vi "scanToString.vi"(0 "instrument handle":refnum<k15>, 1 "wfm info":T3(array[cluster]), 2 "Immediate Trigger Received":bool, 4 "Channels and coupling":T1, 5 "wfm":i8[][](array[numeric]), 9 "Triger Source":i32, 11 "error in":errorcluster {"code" format="%.0x"}, 12 "Trigger Received":bool, 14 "Measurements":T2) -> (3 "instrument handle out":refnum<k15>, 8 "Response String":string, 15 "error out":errorcluster {"code" format="%.0x"})   [LabVIEW 2011]
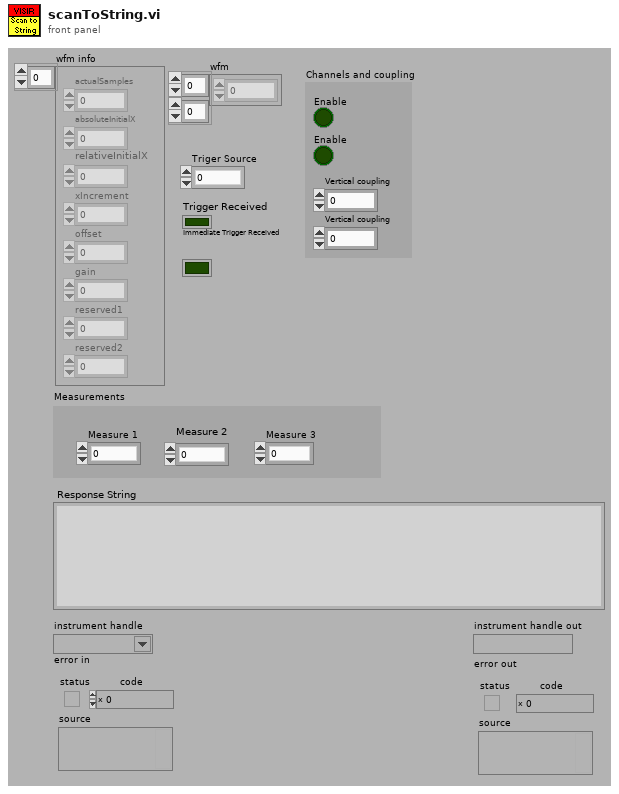
[diagram p1: front panel]
types:
  T1 = cluster{cluster{"Enable":bool, "Enable":bool}, cluster{"Vertical coupling":dbl, "Vertical coupling":dbl}}
  T2 = cluster{"Measure 1":dbl, "Measure 2":dbl, "Measure 3":dbl}
  T3 = cluster{"actualSamples":i32, "absoluteInitialX":dbl, "relativeInitialX":dbl, "xIncrement":dbl, "offset":dbl, "gain":dbl, "reserved1":dbl, "reserved2":dbl}[]
  T4 = cluster{"Vertical coupling":dbl, "Vertical coupling":dbl}
  T5 = cluster{"actualSamples":i32, "absoluteInitialX":dbl, "relativeInitialX":dbl, "xIncrement":dbl, "offset":dbl, "gain":dbl, "reserved1":dbl, "reserved2":dbl}
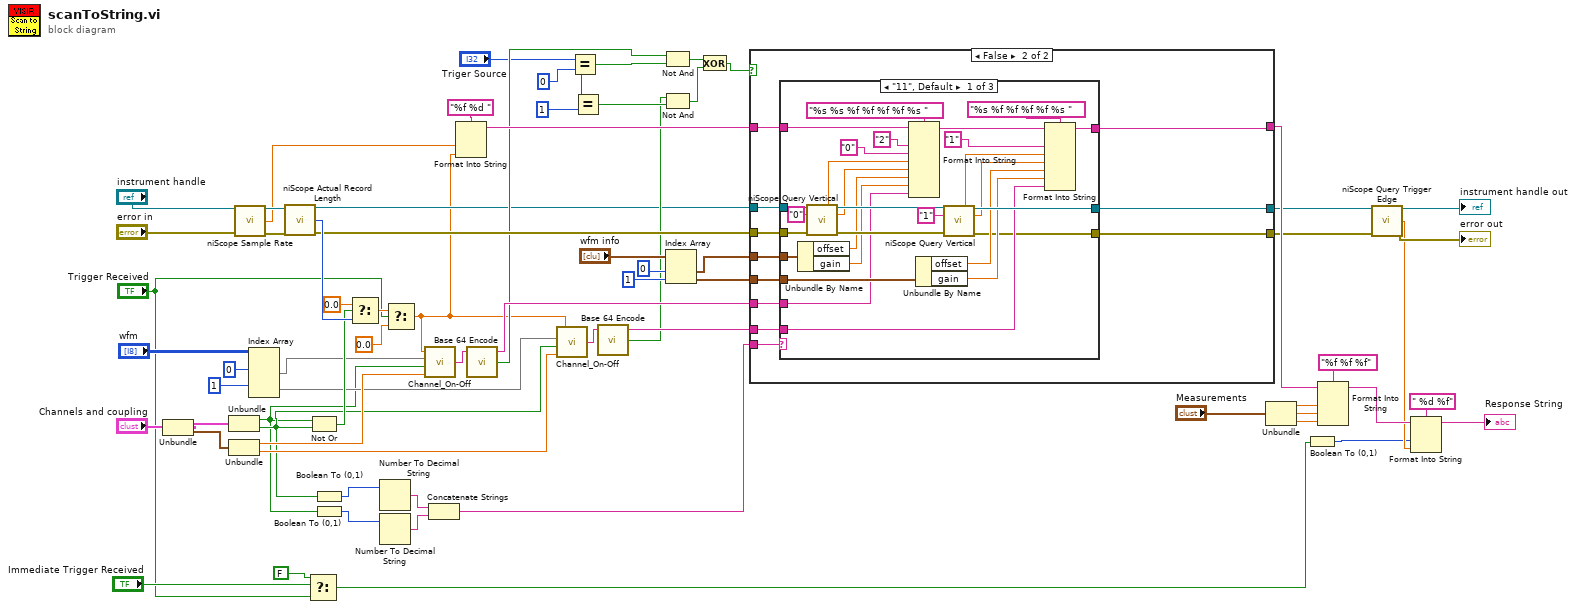
[diagram p0: block diagram]
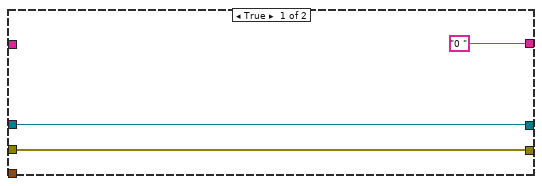
[diagram p2: hidden frame]
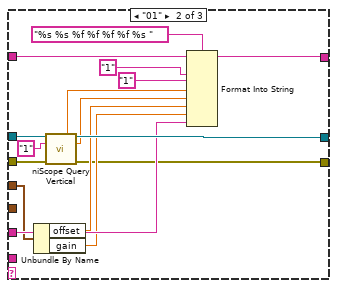
[diagram p3: hidden frame]
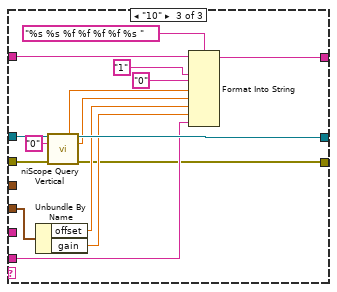
[diagram p4: hidden frame]
diagram:
  n1 = Unbundle("Channels and coupling") -> (w54:cluster{"Enable":bool, "Enable":bool}, w53:T4)
  n2 = Unbundle(w54) -> ("Enable"=w15:bool, "Enable"=w16:bool)
  n3 = Unbundle(w53) -> ("Vertical coupling"=w52:dbl, "Vertical coupling"=w51:dbl)
  n4 = call <instrlib>:"niScope Sample Rate.vi"("instrument handle"="instrument handle", "error in"="error in") -> ("instrument handle out"=w50:refnum<k15>, "actual sample rate"=w49:dbl, "error out"=w48:errorcluster)  [unwired: 11 in]
  n5 = Index Array(array="wfm", index (row) #1=0 ("index (row)"), index (row) #2=1 ("index (row)")) -> (element #1=w40:i8[], element #2=w39:i8[])  [unwired: 2 in]
  n6 = call <instrlib>:"niScope Actual Record Length.vi"("instrument handle"=w50, "error in"=w48) -> ("instrument handle out"=w17:refnum<k15>, "actual record length"=w42:i32, "error out"=w23:errorcluster)  [unwired: 11 in]
  n7 = Select(t=FALSE, s="Immediate Trigger Received", f="Trigger Received") -> (s? t:f=w1:bool)
  n8 = Not Or(1:w16, 2:w15) -> (0:w41:bool)
  n9 = Boolean To (0,1)(Boolean=w16) -> (0, 1=w14:i16)
  n10 = Boolean To (0,1)(Boolean=w15) -> (0, 1=w13:i16)
  n11 = Select(t=0.0, s=w41, f=w42) -> (s? t:f=w9:dbl)
  n12 = Number To Decimal String(number=w14) -> (decimal integer string=w12:string)  [unwired: 1 in]
  n13 = Number To Decimal String(number=w13) -> (decimal integer string=w11:string)  [unwired: 1 in]
  n14 = Select(t=w9, s="Trigger Received", f=0.0 ("t")) -> (s? t:f=w7:dbl)
  n15 = call "Channel_On-Off.vi"("Vertical coupling"=w52, "Enable"=w15, "wfm"=w40, "actual record length"=w7) -> ("String"=w38:string)
  n16 = Concatenate Strings(w12, w11) -> (w10:string)
  n17 = Format Into String(format string="%f %d ", w49, w7) -> (resulting string=w28:string)  [unwired: 2 in, 1 out]
  n18 = call "Base 64 Encode.vi"("Input String"=w38) -> (1:w19:bool, "Output String"=w21:string)  [unwired: 3 in]
  n19 = call "Channel_On-Off.vi"("Vertical coupling"=w51, "Enable"=w16, "wfm"=w39, "actual record length"=w7) -> ("String"=w37:string)
  n20 = Equal?(x="Triger Source", y=0) -> (x = y?=w34:bool)
  n21 = Equal?(x="Triger Source", y=1) -> (x = y?=w30:bool)
  n22 = call "Base 64 Encode.vi"("Input String"=w37) -> (1:w18:bool, "Output String"=w20:string)  [unwired: 3 in]
  n23 = Not And(1:w34, 2:w19) -> (0:w32:bool)
  n24 = Not And(1:w30, 2:w18) -> (0:w29:bool)
  n25 = Index Array(array="wfm info", index #1=0 ("index (row)"), index #2=1 ("index (row)")) -> (element #1=w26:T5, element #2=w25:T5)
  n26 = Exclusive Or(1:w29, 2:w32) -> (0:w31:bool)
  n27 = case shown="False" w31 {
    tunnel: w10 -> [_ w84]
    tunnel: w28 -> [_ w83]
    tunnel: w17 -> [w73 w82]
    tunnel: w23 -> [w71 w81]
    tunnel: [w73 w80] -> w24
    tunnel: w26 -> [_ w79]
    tunnel: w25 -> [_ w78]
    tunnel: w21 -> [_ w77]
    tunnel: w20 -> [_ w76]
    tunnel: ["0 " w75] -> w27
    tunnel: [w71 w74] -> w22
    frame True {
    }
    frame False {
      n28 = case shown="\"11\", Default" w84 {
        tunnel: w83 -> [w110 w127 w143]
        tunnel: [w102 w126 w139] -> w75
        tunnel: w77 -> [w97 w124 _]
        tunnel: w76 -> [w100 _ w137]
        tunnel: w82 -> [w111 w122 w144]
        tunnel: w81 -> [w106 w123 w142]
        tunnel: [w101 w125 w138] -> w80
        tunnel: w79 -> [w99 w121 _]
        tunnel: w78 -> [w98 _ w140]
        tunnel: [w85 w113 w129] -> w74
        frame "11", Default {
          n29 = Unbundle By Name(w99) -> ("offset"=w95:dbl, "gain"=w96:dbl)
          n30 = call "niScope Query Vertical.vi"("instrument handle"=w111, "channel name"="0", "error in"=w106) -> ("probe attenuation"=w93:dbl, "instrument handle out"=w107:refnum<k15>, "vertical range"=w94:dbl, "error out"=w105:errorcluster)  [unwired: 5 in, 4 out]
          n31 = Format Into String(format string="%s %s %f %f %f %f %s ", initial string=w110, "2", "0", w93, w94, w95, w96, w97) -> (resulting string=w108:string)  [unwired: 1 in, 1 out]
          n32 = Unbundle By Name(w98) -> ("offset"=w89:dbl, "gain"=w90:dbl)
          n33 = call "niScope Query Vertical.vi"("instrument handle"=w107, "channel name"="1", "error in"=w105) -> ("probe attenuation"=w87:dbl, "instrument handle out"=w101:refnum<k15>, "vertical range"=w88:dbl, "error out"=w85:errorcluster)  [unwired: 5 in, 4 out]
          n34 = Format Into String(format string="%s %f %f %f %f %s ", initial string=w108, "1", w87, w88, w89, w90, w100) -> (resulting string=w102:string)  [unwired: 1 in, 1 out]
        }
        frame "01" {
          n35 = Unbundle By Name(w121) -> ("offset"=w118:dbl, "gain"=w119:dbl)
          n36 = call "niScope Query Vertical.vi"("instrument handle"=w122, "channel name"="1", "error in"=w123) -> ("probe attenuation"=w116:dbl, "instrument handle out"=w125:refnum<k15>, "vertical range"=w117:dbl, "error out"=w113:errorcluster)  [unwired: 5 in, 4 out]
          n37 = Format Into String(format string="%s %s %f %f %f %f %s ", initial string=w127, "1", "1", w116, w117, w118, w119, w124) -> (resulting string=w126:string)  [unwired: 1 in, 1 out]
        }
        frame "10" {
          n38 = Unbundle By Name(w140) -> ("offset"=w134:dbl, "gain"=w135:dbl)
          n39 = call "niScope Query Vertical.vi"("instrument handle"=w144, "channel name"="0", "error in"=w142) -> ("probe attenuation"=w132:dbl, "instrument handle out"=w138:refnum<k15>, "vertical range"=w133:dbl, "error out"=w129:errorcluster)  [unwired: 5 in, 4 out]
          n40 = Format Into String(format string="%s %s %f %f %f %f %s ", initial string=w143, "1", "0", w132, w133, w134, w135, w137) -> (resulting string=w139:string)  [unwired: 1 in, 1 out]
        }
      }
    }
  }
  n41 = Unbundle("Measurements") -> ("Measure 1"=w58:dbl, "Measure 2"=w56:dbl, "Measure 3"=w57:dbl)
  n42 = Boolean To (0,1)(Boolean=w1) -> (0, 1=w5:i16)
  n43 = Format Into String(format string="%f %f %f", initial string=w27, w58, w56, w57) -> (resulting string=w64:string)  [unwired: 1 in, 1 out]
  n44 = call "niScope Query Trigger Edge.vi"("instrument handle"=w24, "error in"=w22) -> ("instrument handle out"=→"instrument handle out":refnum<k15>, "trigger level"=w44:dbl, "error out"=→"error out":errorcluster)  [unwired: 6 in, 5 out]
  n45 = Format Into String(format string=" %d %f", initial string=w64, w5, w44) -> (resulting string=→"Response String":string)  [unwired: 1 in, 1 out]
